vi "Read DCM Ref.vi"(8 "error in (no error)":errorcluster, 11 "DCM-DSI-HW in":refnum<class "DCM-DSI.lvclass">) -> (0 "error out":errorcluster, 2 "DCM Ref":refnum<class "DCM - RT.lvclass">, 3 "DCM-DSI-HW out":refnum<class "DCM-DSI.lvclass">)   [LabVIEW 2016, in "DCM-DSI.lvclass"]
uses:
  DCM-DSI.lvclass
  <vilib>/Powertrain Controls/Device Drivers/DCM/Rev0/RT/DCM - RT.lvclass
  DCM-DSI.lvclass/DCM-DSI.ctl
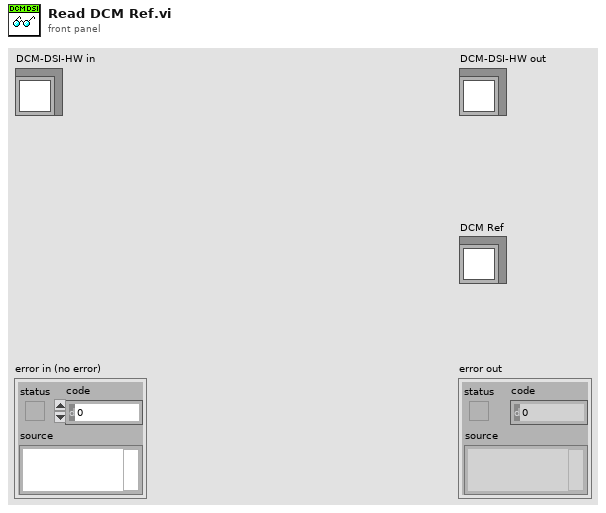
[diagram p1: front panel]
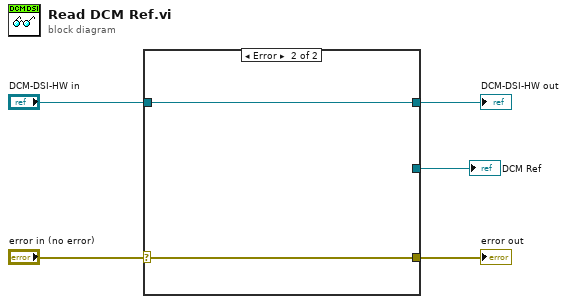
[diagram p0: block diagram]
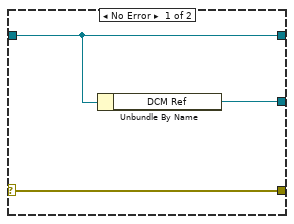
[diagram p2: hidden frame]
diagram:
  n1 = case shown="Error" "error in (no error)" {
    selector: "error in (no error)" -> [w6 w9]
    tunnel: "DCM-DSI-HW in" -> [w7 w10]
    tunnel: [w8 _] -> w4
    tunnel: [w7 w10] -> w2
    tunnel: [w6 w9] -> w1
    frame No Error {
      n2 = Unbundle By Name(w7) -> ("DCM Ref"=w8:refnum<class "DCM - RT.lvclass">)
    }
    frame Error {
    }
  }
  "error out" <- w1
  "DCM-DSI-HW out" <- w2
  "DCM Ref" <- w4
